vi "Arrrys and For loops.vi"() -> ()   [LabVIEW 2024]
panel:
  out "Array":dbl[](array[numeric])
  out "Shift Register Val":dbl
  out "Numeric":dbl
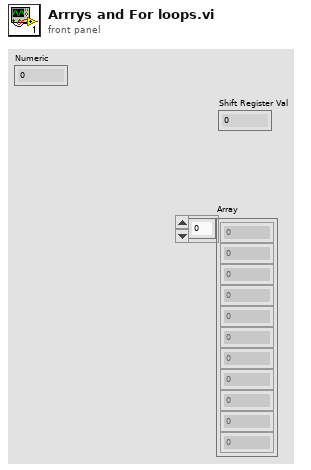
[diagram p1: front panel]
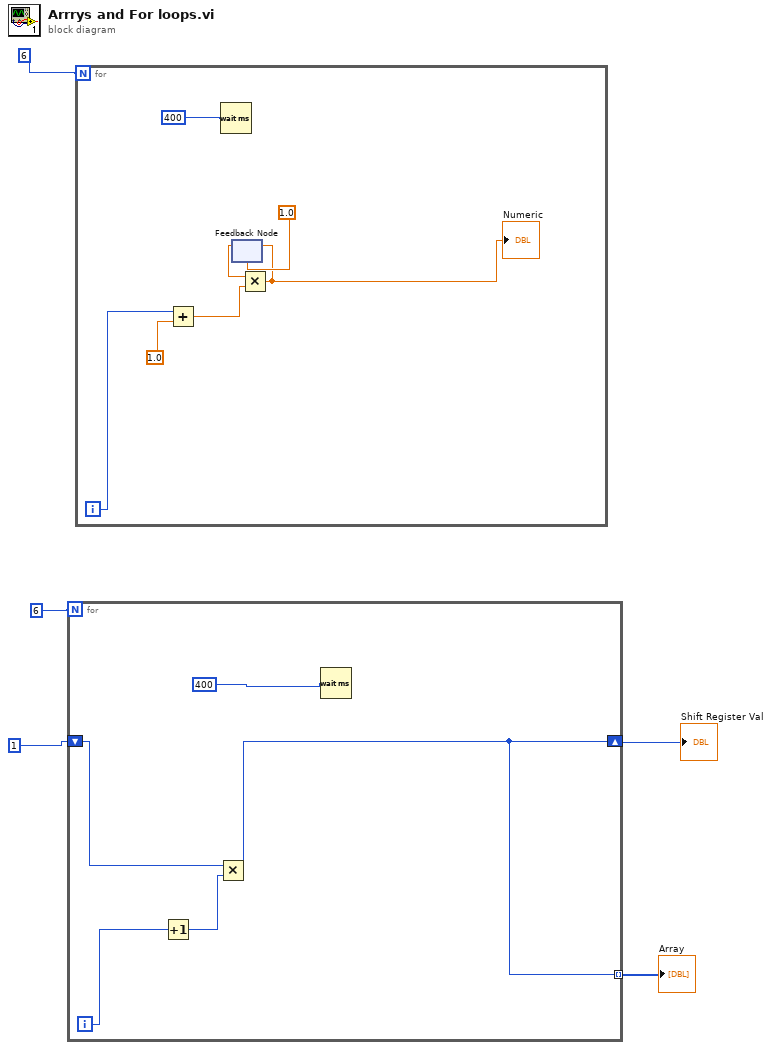
[diagram p0: block diagram]
diagram:
  n1 = for {
    N: 6 -> [_]
    shift-right: [w6] -> w4
    shift-left: 1 -> [w8]
    tunnel: [w6] -> w1 mode=indexing
    i -> [w10]
    n2 = Increment(x=w10) -> (x+1=w9:i32)
    n3 = Multiply(x=w8, y=w9) -> (x*y=w6:i32)
    n4 = Wait (ms)(milliseconds to wait=u32 400) -> ()  [unwired: 1 out]
  }
  "Shift Register Val" <- w4
  "Array" <- w1
  n5 = for {
    N: 6 -> [_]
    i -> [w16]
    n6 = Add(x=w16, y=1.0) -> (x+y=w15:dbl)
    n7 = Wait (ms)(milliseconds to wait=u32 400) -> ()  [unwired: 1 out]
    n8 = feedback #1(1.0) -> (w14:dbl)
    n9 = Multiply(x=w14, y=w15) -> (x*y=w12:dbl)
    "Numeric" <- w12
    n10 = feedback-in #1(w12) -> ()
  }
